vi "SP_Breakdown Summery DayWisewise.vi"() -> ()   [LabVIEW 2017]
uses:
  <vilib>/Math Plots/3D Math Plots/3D Pie/3D Pie XCtrl/3D Pie.xctl
  <vilib>/addons/database/Connection.llb/DB Tools Open Connec (Path).vi
  <vilib>/Math Plots/3D Math Plots/3D Pie/3D Pie Datatype/Public/Plot Helper (Vector).vi
  <vilib>/addons/database/NI_Database_API.lvlib
  <vilib>/Math Plots/3D Math Plots/3D Pie/3D Pie Datatype/3D Pie Datatype.lvclass
panel:
  out "error out 2":errorcluster
  out "Boolean":bool
  in  "Cancel Button - Archive":bool
  in  "Get Rport 2":bool
  in  "Download 2":bool
  in  "error in":errorcluster
  in  "To":timestamp format="%<%Y-%m-%d>T"
  in  "From":timestamp format="%<%Y-%m-%d>T"
  out "error out":errorcluster
  out "O/P 4":string[](array[string])
  out "month":string
  out "Count":string[](array[string])
  out "Station ID":string[](array[string])
  out "Count out":string[](array[string])
  out "Elements Found out":string[](array[string])
  in  "stop":bool
  in  "Select Station":string(combo)
  in  "Shift":string(combo)
  out "T":string
  out "SS":string
  out "Q":string
  out "Maint":string
  out "Mat":string
  out "S":string
  in  "Select Year":string(combo)
  in  "Select Month":string(combo)
  in  "Tab Control":T1(tab)
  out "Table Control":string[][](table)
  out "heading 6":string="Total"
  out "heading 5":string="Production"
  out "heading 4":string="Qaulity"
  out "heading 3":string="Maintenance"
  out "heading2":string="Logistics"
  out "heading 1":string="Gap Leader"
  out "Count":refnum<class "3D Plot Datatype.lvclass">[](xcontrol)
  out "Duration":refnum<class "3D Plot Datatype.lvclass">[](xcontrol)
  # "Breakdown Summary Report (Day Wise)"
  # "S"
  # "M"
  # "TT"
  # "M"
  # "Q"
  # "SS"
  # "Designed And Developed By - Infinity Automation Systems Pvt. Ltd."
  # "Material"
  # "Date"
  # "Maintenance"
  # "Quality"
  # "Startup/Setup"
  # "Total"
  # "Safety"
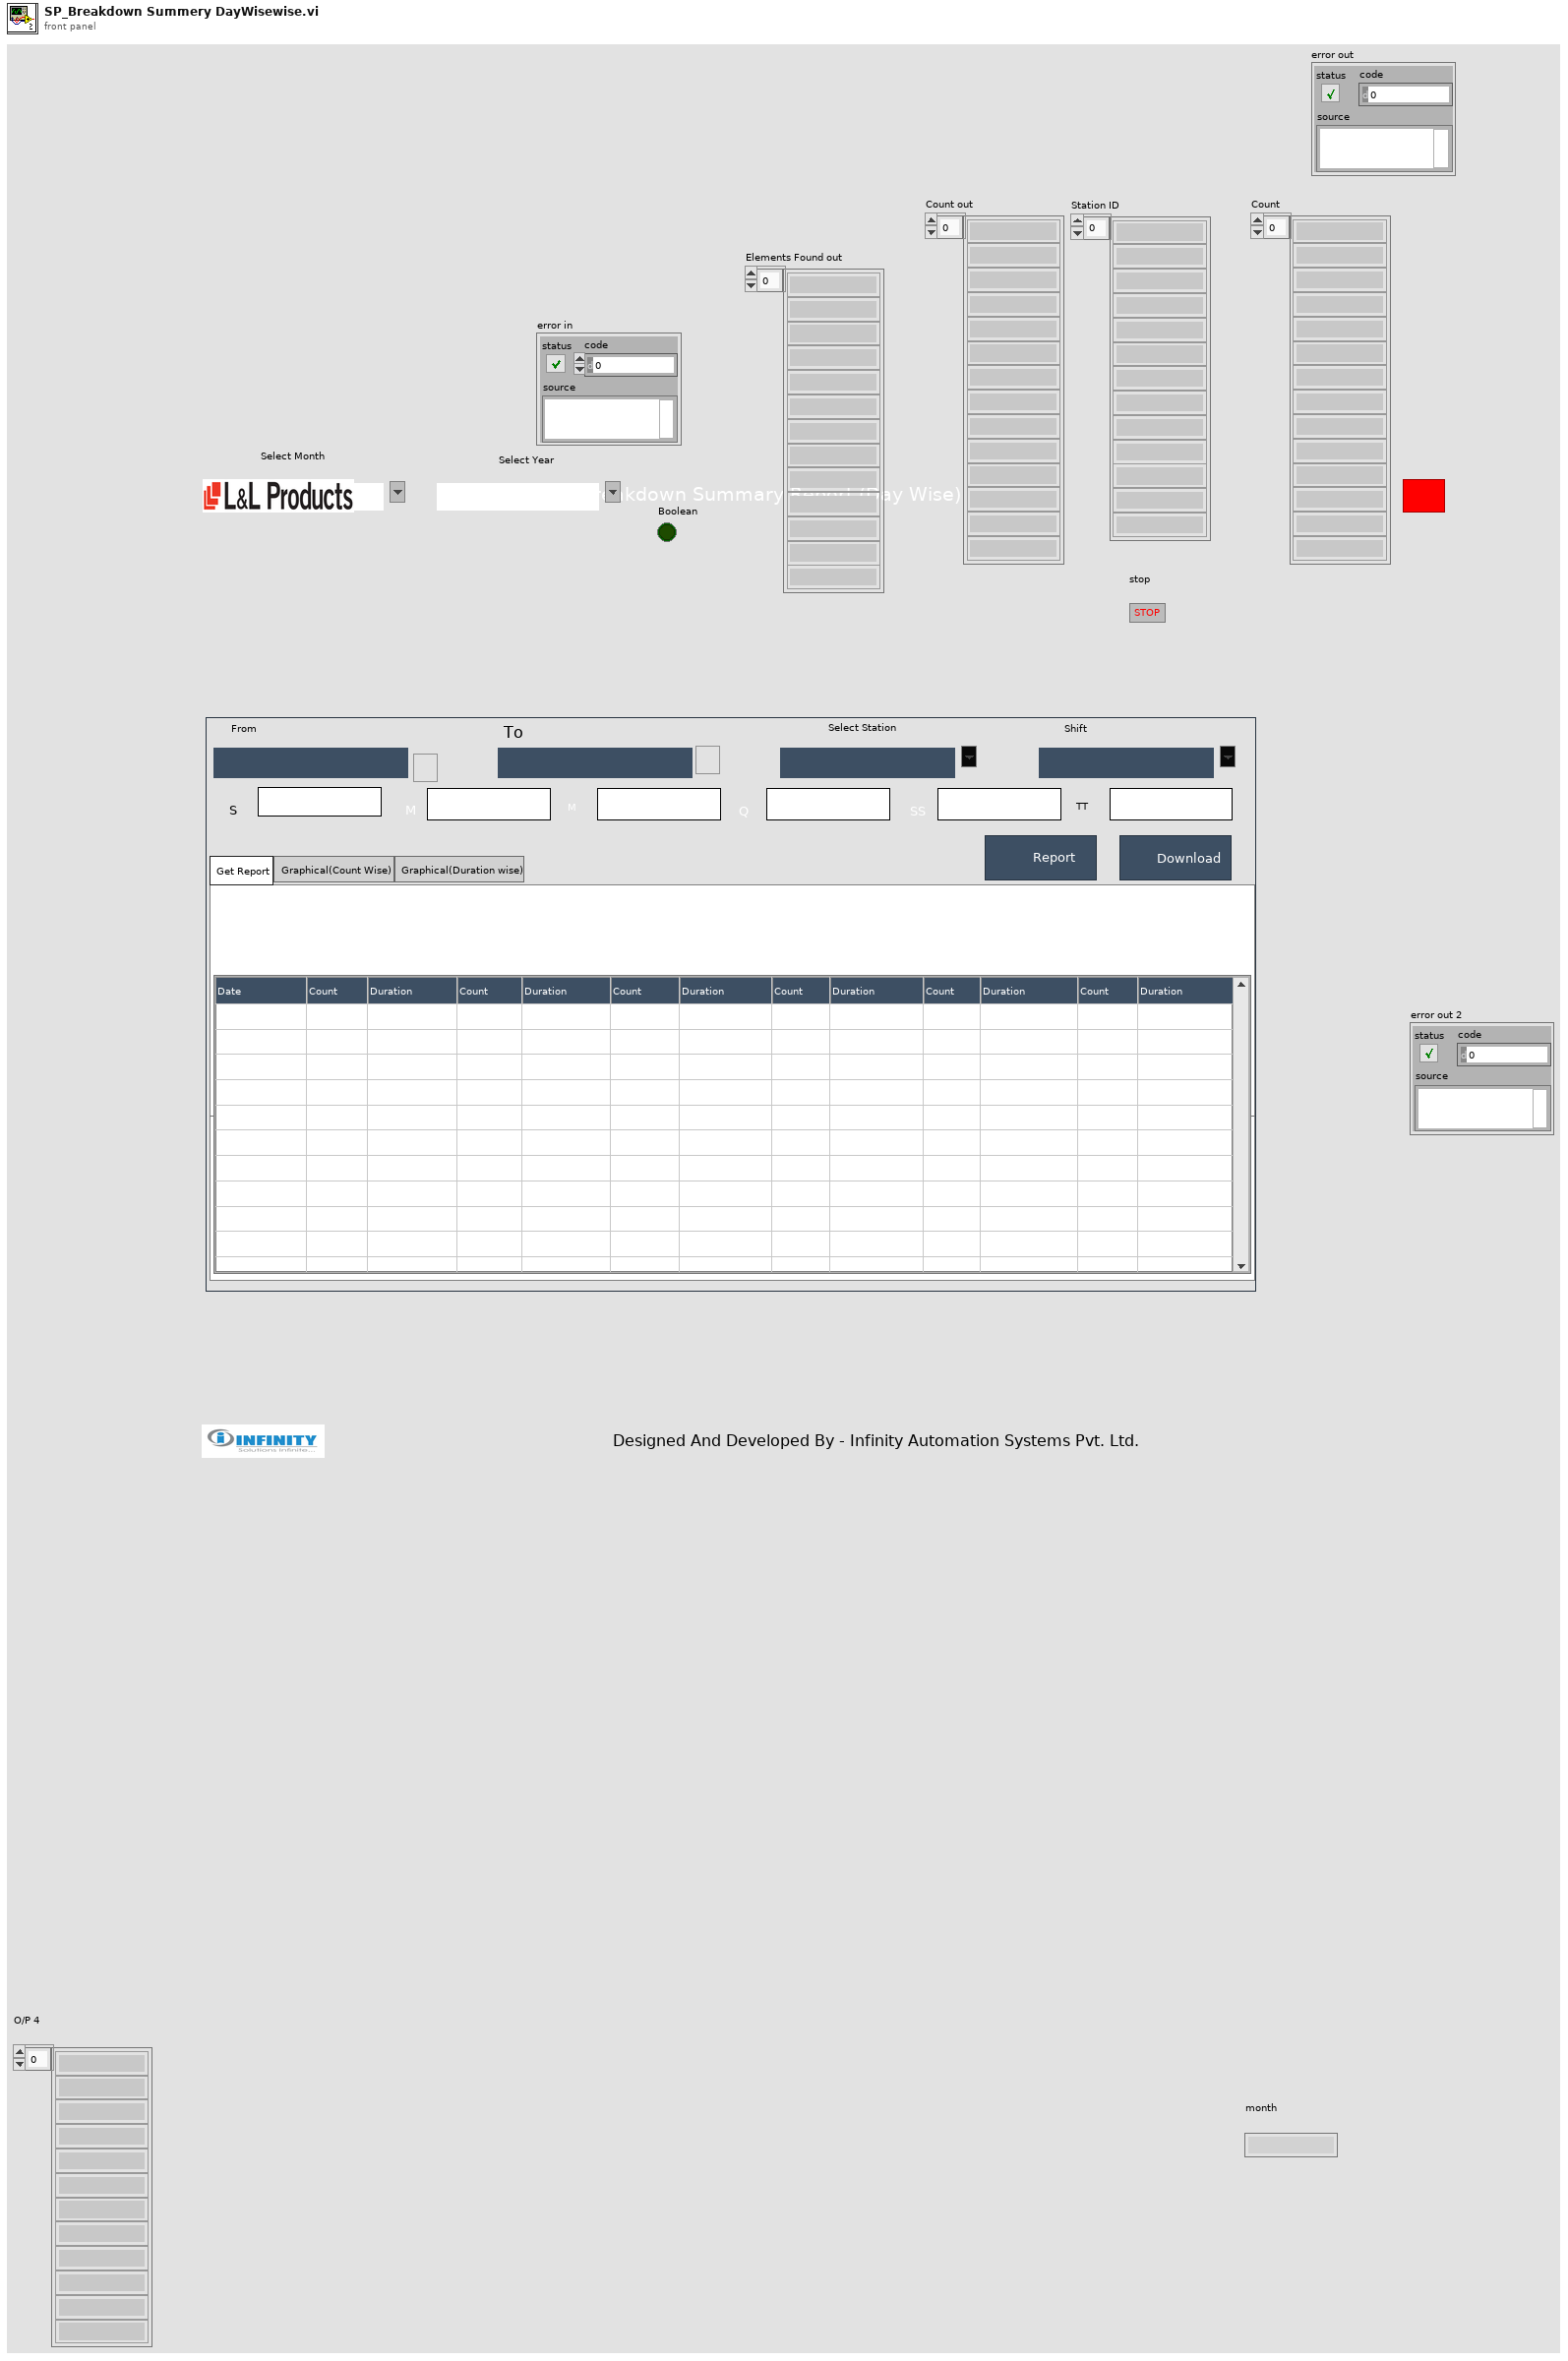
[diagram p1: front panel]
types:
  T1 = enum32{"Get Report", "Graphical(Count Wise) ", "Graphical(Duration wise)"}
  T2 = typedef "NI_Database_API.lvlib/Conn ObjectReference.ctl" = refnum<k1>
  T3 = enum32{"invalid app kind", "Development System", "Run Time System", "Student Edition", "Embedded LabVIEW", "Evaluation", "Custom"}
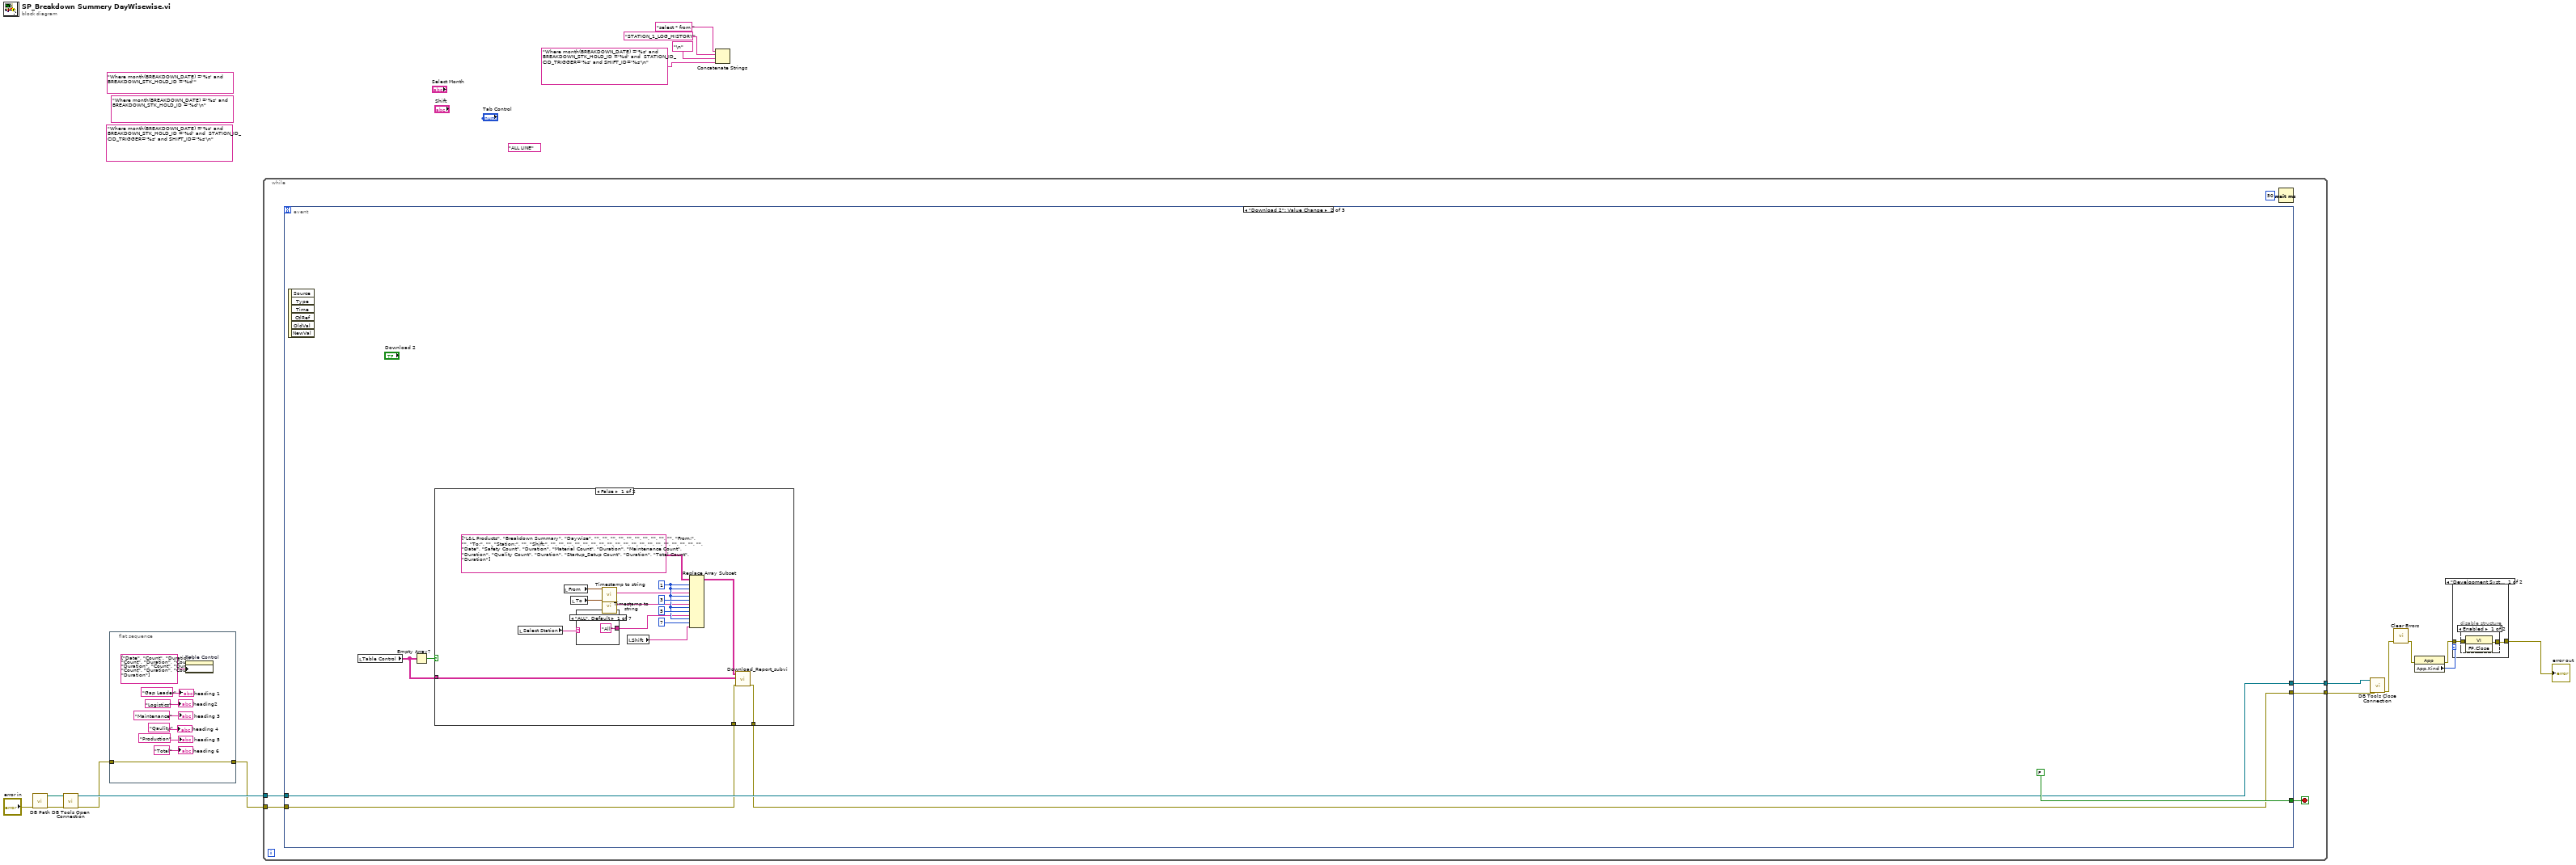
[diagram p0: block diagram]
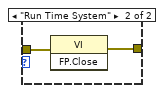
[diagram p3: hidden frame]
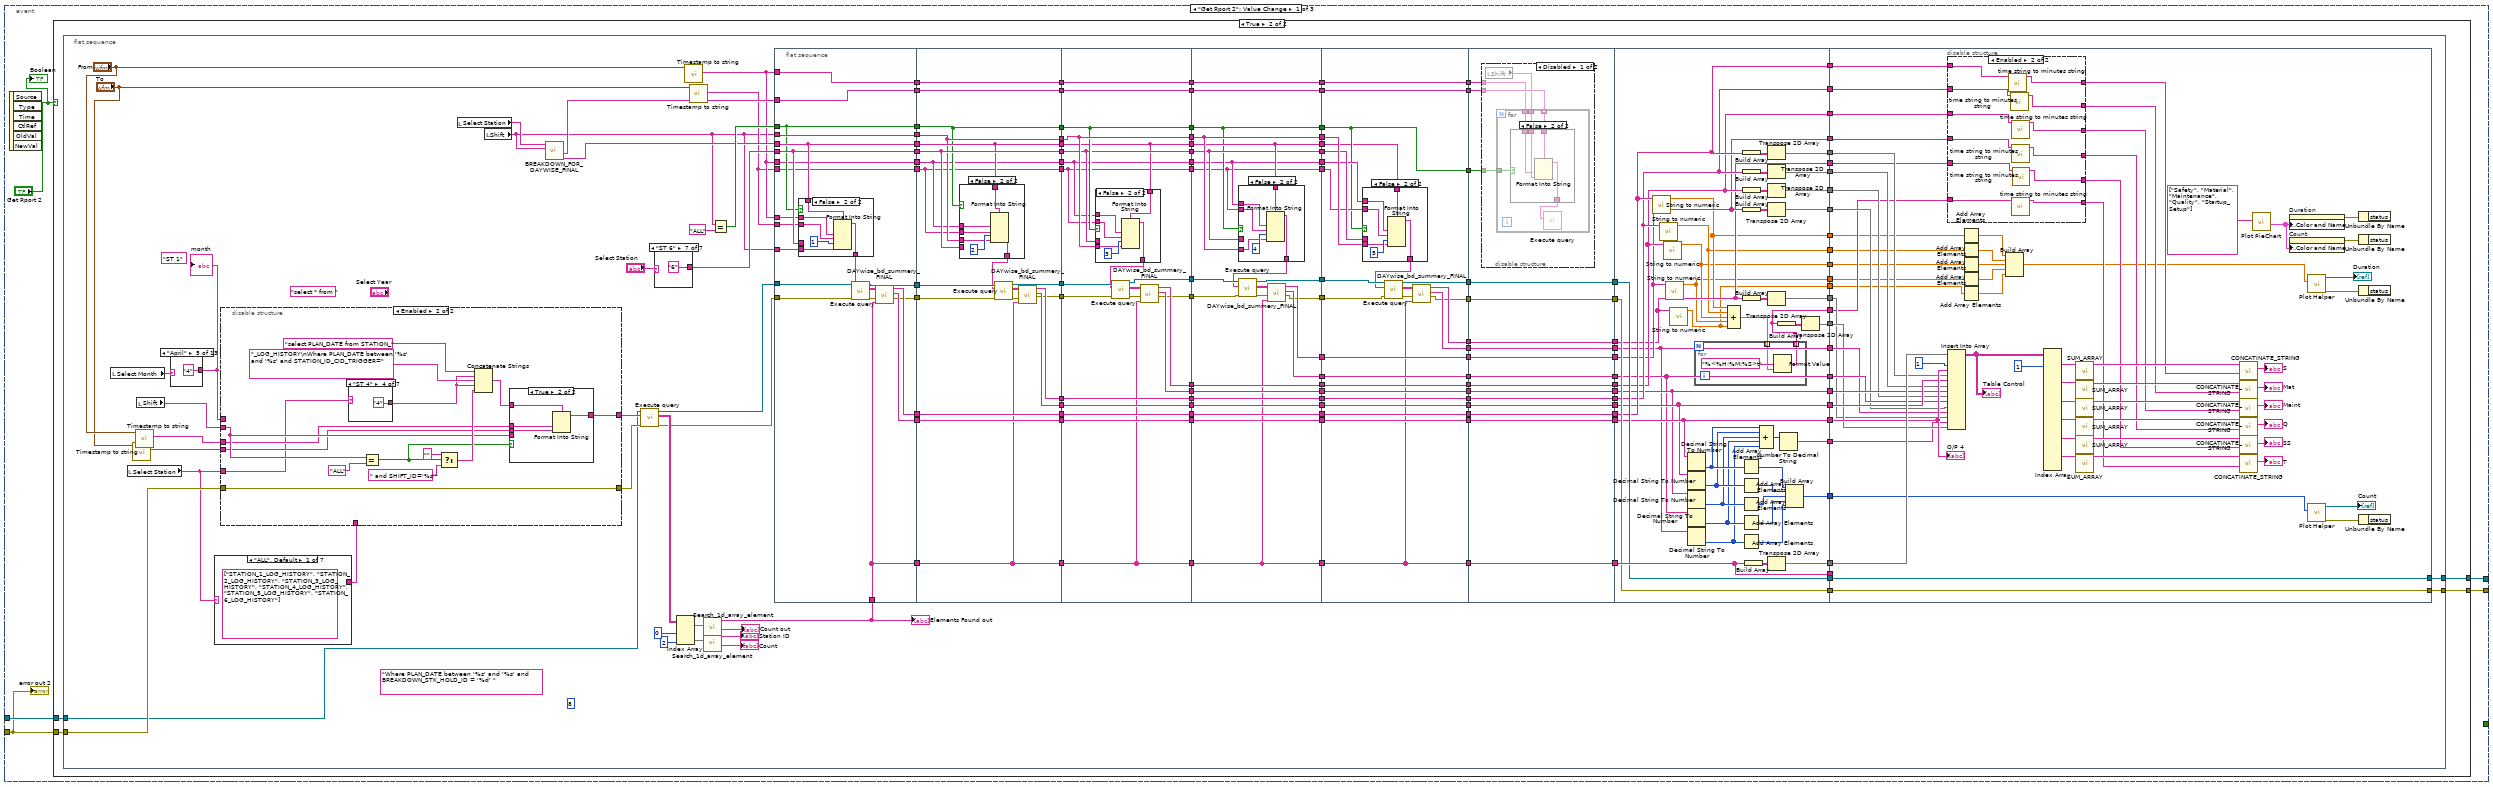
[diagram p4: hidden frame]
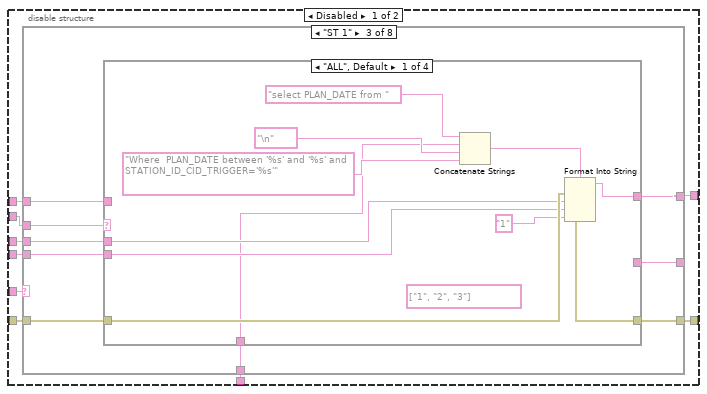
[diagram p6: hidden frame]
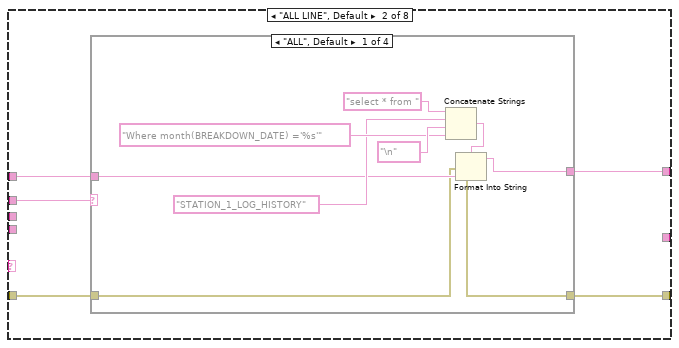
[diagram p8: hidden frame]
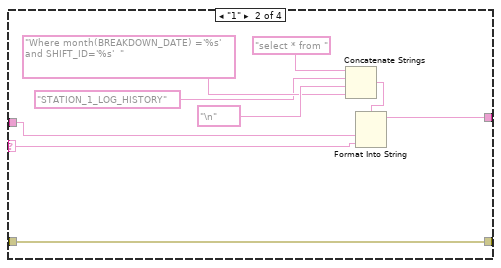
[diagram p9: hidden frame]
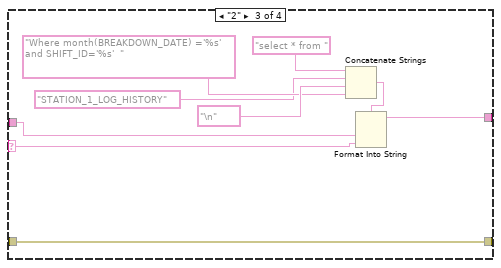
[diagram p10: hidden frame]
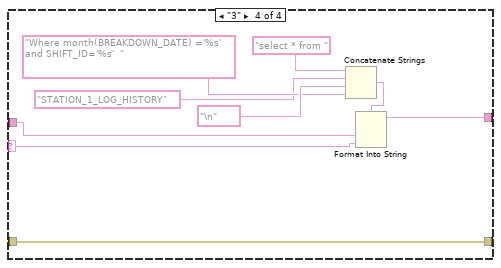
[diagram p11: hidden frame]
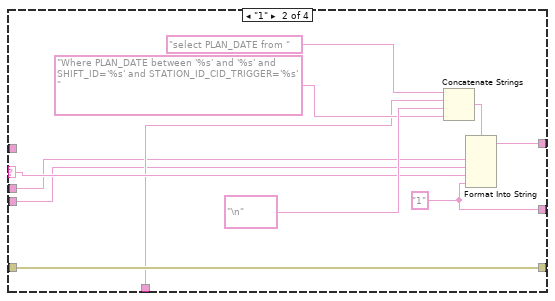
[diagram p12: hidden frame]
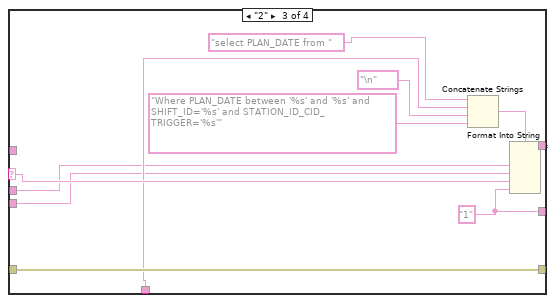
[diagram p13: hidden frame]
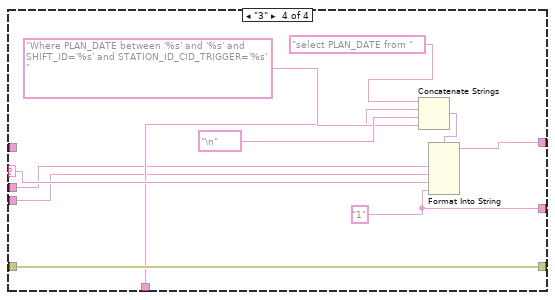
[diagram p14: hidden frame]
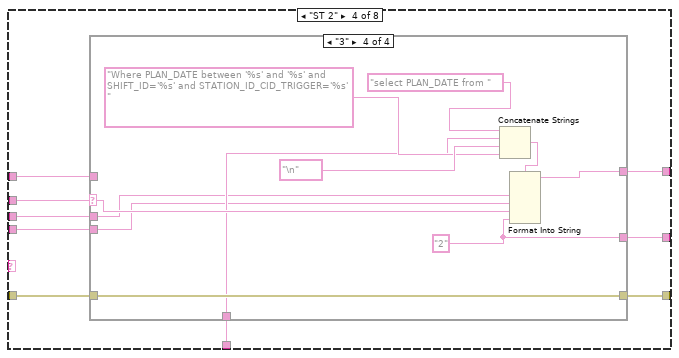
[diagram p15: hidden frame]
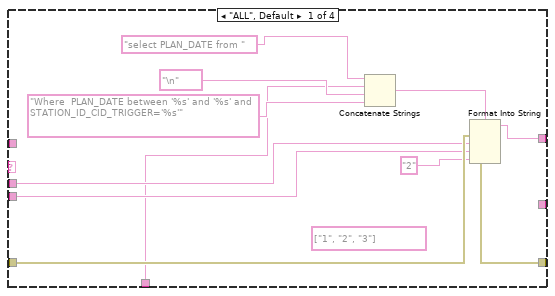
[diagram p16: hidden frame]
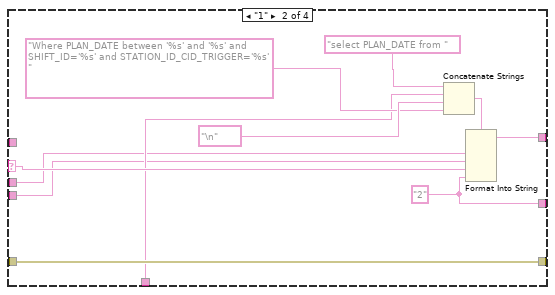
[diagram p17: hidden frame]
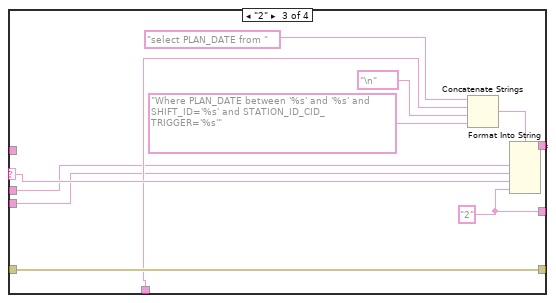
[diagram p18: hidden frame]
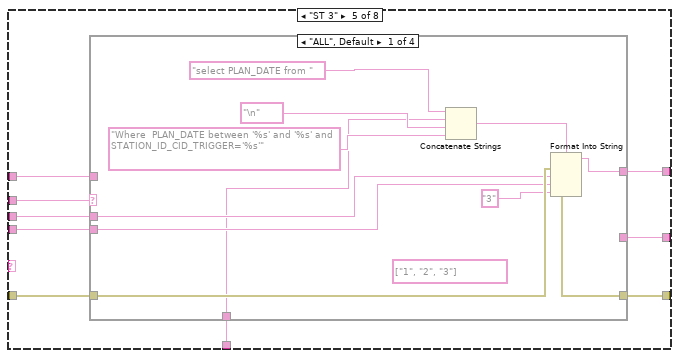
[diagram p19: hidden frame]
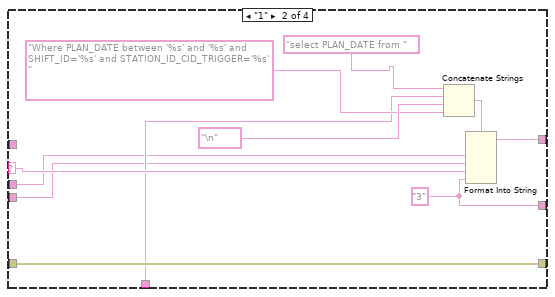
[diagram p20: hidden frame]
diagram:
  (unwired) "Where month(BREAKDOWN_DATE) ='%s' and  BREAKDOWN_STK_HOLD_ID ='%d' and  STATION_ID_CID_TRIGGER='%s' and SHIFT_ID='%s'\n" ("condition")
  (unwired) "Where month(BREAKDOWN_DATE) ='%s' and  BREAKDOWN_STK_HOLD_ID ='%d'" ("condition")
  (unwired) "Where month(BREAKDOWN_DATE) ='%s' and  BREAKDOWN_STK_HOLD_ID ='%d'\n" ("condition")
  (unwired) "ALL LINE" ("Select Line 2")
  n1 = call "DB Path.vi"("error in"="error in") -> ("error out"=w17:errorcluster, "DB Path"=w16:path)  [unwired: 9 in]
  n2 = call-poly <vilib>:"DB Tools Open Connection.vi"("error in (no error)"=w17, "connection information"=w16) -> ("error out"=w2:errorcluster, "connection reference"=w15:T2)  [unwired: 6 in]
  n3 = flat-sequence {
    tunnel: [w18] -> w1
    tunnel: w2 -> [w18]
    frame #0 {
      n4 = property on="Table Control" class="Tbl (strict)"("Column Headers[]"=string[] ["Date", "Count", "Duration", "Count", "Duration", "Count", "Duration", "Count", "Duration", "Count", "Duration", "Count", "Duration"] ("Column Header Strings[]")) -> ()  [unwired: 2 in, 2 out]
      "heading 1" <- "Gap Leader" ("heading 1")
      "heading2" <- "Logistics" ("heading2")
      "heading 3" <- "Maintenance" ("heading 3")
      "heading 4" <- "Qaulity" ("heading 4")
      "heading 5" <- "Production" ("heading 5")
      "heading 6" <- "Total" ("heading 6")
    }
  }
  n5 = while {
    tunnel: w1 -> [w31]
    tunnel: w15 -> [w30]
    tunnel: [w28] -> w5
    tunnel: [w27] -> w6
    stop <- w29 stop-if-true
    n6 = event shown="[1] \"Download 2\": Value Change" {
      selector: _ -> [_ _ _]
      dyn-events: _ -> [_ _ _]
      timeout: _ -> [_ _ _]
      tunnel: w31 -> [w33 w985 w1014]
      tunnel: w30 -> [w36 w986 w1013]
      tunnel: [_ FALSE ("Cancel Button - Archive") "Cancel Button - Archive"] -> w29
      tunnel: [w35 w984 w1014] -> w28
      tunnel: [w34 w986 w1013] -> w27
      event "Get Rport 2": Value Change {
        n7 = event-data() -> ()  [unwired: 1 in, 6 out]
        n8 = case shown="True" "Get Rport 2" {
          tunnel: w33 -> [_ w40]
          tunnel: w36 -> [_ w39]
          tunnel: [_ w38] -> w35
          tunnel: [_ w37] -> w34
          frame False {
          }
          frame True {
            n9 = flat-sequence {
              tunnel: w40 -> [w193]
              tunnel: w39 -> [w120]
              tunnel: [w118] -> w38
              tunnel: [w116] -> w37
              frame #0 {
                (unwired) "select * from " ("string")
                (unwired) 8 ("disabled index (col)")
                (unwired) "Where PLAN_DATE between '%s' and '%s' and BREAKDOWN_STK_HOLD_ID = '%d' "
                (unwired) "ST 1" ("Select Station")
                n10 = local read "Select Month"() -> (w190:string)
                n11 = local read "Select Station"() -> (w112:string)
                n12 = call "Timestamp to string.vi"("time stamp"="To") -> ("Date"=w52:string)  [unwired: 8 in, 2 out]
                n13 = call "Timestamp to string.vi"("time stamp"="From") -> ("Date"=w53:string)  [unwired: 8 in, 2 out]
                n14 = local read "Shift"() -> (w100:string)
                n15 = case shown="\"April\"" w190 {
                  tunnel: ["1" "1" "2" "3" "4" "5" "6" "7" "8" "9" "10" "11" "12"] -> w119
                  frame "False", Default {
                  }
                  frame "January" {
                  }
                  frame "February" {
                  }
                  frame "March" {
                  }
                  frame "April" {
                  }
                  frame "May" {
                  }
                  frame "June" {
                  }
                  frame "July" {
                  }
                  frame "August" {
                  }
                  frame "September" {
                  }
                  frame "October" {
                  }
                  frame "November" {
                  }
                  frame "December" {
                  }
                }
                "month" <- w119
                n16 = case shown="\"ALL\", Default" w112 {
                  tunnel: [_ "STATION_1_LOG_HISTORY" "STATION_2_LOG_HISTORY" ("table") "STATION_3_LOG_HISTORY" ("table") "STATION_4_LOG_HISTORY" ("table") "STATION_5_LOG_HISTORY" ("table") "STATION_6_LOG_HISTORY" ("table")] -> w99
                  frame "ALL", Default {
                    (unwired) string[] ["STATION_1_LOG_HISTORY", "STATION_2_LOG_HISTORY", "STATION_3_LOG_HISTORY", "STATION_4_LOG_HISTORY", "STATION_5_LOG_HISTORY", "STATION_6_LOG_HISTORY"]
                  }
                  frame "ST 1" {
                  }
                  frame "ST 2" {
                  }
                  frame "ST 3" {
                  }
                  frame "ST 4" {
                  }
                  frame "ST 5" {
                  }
                  frame "ST 6" {
                  }
                }
                n17 = disable-structure shown="Enabled" {
                  disable-tunnel: [w206 w571] -> w197
                  disable-tunnel: w193 -> [w205 w567]
                  disable-tunnel: [w204 w567] -> w192
                  disable-tunnel: w119 -> [w203 _]
                  disable-tunnel: w112 -> [w202 w566]
                  disable-tunnel: w100 -> [w201 w570]
                  disable-tunnel: w99 -> [w200 _]
                  disable-tunnel: w53 -> [w199 w569]
                  disable-tunnel: w52 -> [w198 w568]
                  frame Disabled {
                    n18 = case shown="\"ST 1\"" w202 {
                      tunnel: w203 -> [_ w211 w256 w309 w362 w415 w468 w521]
                      tunnel: [_ w210 w255 w308 w361 w414 w467 w520] -> w206
                      tunnel: w205 -> [_ w209 w254 w307 w360 w413 w466 w519]
                      tunnel: [_ w208 w253 w306 w359 w412 w465 w518] -> w204
                      tunnel: [_ _ w252 w305 w358 w411 w464 w517] -> _
                      tunnel: w199 -> [_ _ w251 w304 w357 w410 w463 w516]
                      tunnel: w198 -> [_ _ w250 w303 w356 w409 w462 w515]
                      tunnel: w201 -> [_ w207 w248 w301 w354 w407 w460 w513]
                      tunnel: w200 -> [_ _ w249 w302 w355 w408 w461 w514]
                      frame "False" {
                      }
                      frame "ALL LINE", Default {
                        n19 = case shown="\"ALL\", Default" w207 {
                          selector: w207 -> [_ w222 w231 w240]
                          tunnel: [w216 w225 w234 w243] -> w210
                          tunnel: [w215 w221 w230 w239] -> w208
                          tunnel: w211 -> [w213 w223 w232 w241]
                          tunnel: w209 -> [w212 w221 w230 w239]
                          frame "ALL", Default {
                            n20 = Concatenate Strings("select * from " ("string"), "STATION_1_LOG_HISTORY" ("table"), "\n" ("string"), "Where month(BREAKDOWN_DATE) ='%s'" ("condition")) -> (w217:string)
                            n21 = Format Into String(format string=w217, error in=w212, w213) -> (resulting string=w216:string, error out=w215:errorcluster)  [unwired: 1 in]
                          }
                          frame "1" {
                            n22 = Concatenate Strings("select * from " ("string"), "STATION_1_LOG_HISTORY" ("table"), "\n" ("string"), "Where month(BREAKDOWN_DATE) ='%s' and SHIFT_ID='%s'  " ("condition")) -> (w227:string)
                            n23 = Format Into String(format string=w227, w223, w222) -> (resulting string=w225:string)  [unwired: 2 in, 1 out]
                          }
                          frame "2" {
                            n24 = Concatenate Strings("select * from " ("string"), "STATION_1_LOG_HISTORY" ("table"), "\n" ("string"), "Where month(BREAKDOWN_DATE) ='%s' and SHIFT_ID='%s'  " ("condition")) -> (w236:string)
                            n25 = Format Into String(format string=w236, w232, w231) -> (resulting string=w234:string)  [unwired: 2 in, 1 out]
                          }
                          frame "3" {
                            n26 = Concatenate Strings("select * from " ("string"), "STATION_1_LOG_HISTORY" ("table"), "\n" ("string"), "Where month(BREAKDOWN_DATE) ='%s' and SHIFT_ID='%s'  " ("condition")) -> (w245:string)
                            n27 = Format Into String(format string=w245, w241, w240) -> (resulting string=w243:string)  [unwired: 2 in, 1 out]
                          }
                        }
                      }
                      frame "ST 1" {
                        n28 = case shown="\"ALL\", Default" w248 {
                          selector: w248 -> [_ w275 w286 w297]
                          tunnel: [w263 w276 w287 w298] -> w255
                          tunnel: [w262 w274 w285 w296] -> w253
                          tunnel: w256 -> [_ _ _ _]
                          tunnel: w254 -> [w261 w274 w285 w296]
                          tunnel: [_ w272 w283 w294] -> w252
                          tunnel: w251 -> [w259 w270 w281 w292]
                          tunnel: w250 -> [w258 w269 w280 w291]
                          tunnel: w249 -> [w257 w271 w282 w293]
                          frame "ALL", Default {
                            (unwired) string[] ["1", "2", "3"]
                            n29 = Concatenate Strings("select PLAN_DATE from " ("string"), w257, "\n" ("string"), "Where  PLAN_DATE between '%s' and '%s' and  STATION_ID_CID_TRIGGER='%s'" ("condition")) -> (w264:string)
                            n30 = Format Into String(format string=w264, error in=w261, w259, w258, "1") -> (resulting string=w263:string, error out=w262:errorcluster)  [unwired: 1 in]
                          }
                          frame "1" {
                            w272 = "1"
                            n31 = Concatenate Strings("select PLAN_DATE from " ("string"), w271, "\n" ("string"), "Where PLAN_DATE between '%s' and '%s' and SHIFT_ID='%s' and STATION_ID_CID_TRIGGER='%s'   " ("condition")) -> (w273:string)
                            n32 = Format Into String(format string=w273, w270, w269, w275, w272) -> (resulting string=w276:string)  [unwired: 2 in, 1 out]
                          }
                          frame "2" {
                            w283 = "1" ("input 3")
                            n33 = Concatenate Strings("select PLAN_DATE from " ("string"), w282, "\n" ("string"), "Where PLAN_DATE between '%s' and '%s' and SHIFT_ID='%s' and STATION_ID_CID_TRIGGER='%s'" ("condition")) -> (w288:string)
                            n34 = Format Into String(format string=w288, w281, w280, w286, w283) -> (resulting string=w287:string)  [unwired: 2 in, 1 out]
                          }
                          frame "3" {
                            w294 = "1" ("input 3")
                            n35 = Concatenate Strings("select PLAN_DATE from " ("string"), w293, "\n" ("string"), "Where PLAN_DATE between '%s' and '%s' and SHIFT_ID='%s' and STATION_ID_CID_TRIGGER='%s'   " ("condition")) -> (w299:string)
                            n36 = Format Into String(format string=w299, w292, w291, w297, w294) -> (resulting string=w298:string)  [unwired: 2 in, 1 out]
                          }
                        }
                      }
                      frame "ST 2" {
                        n37 = case shown="\"3\"" w301 {
                          selector: w301 -> [_ w328 w339 w350]
                          tunnel: [w317 w329 w340 w351] -> w308
                          tunnel: [w316 w327 w338 w349] -> w306
                          tunnel: w309 -> [_ _ _ _]
                          tunnel: w307 -> [w315 w327 w338 w349]
                          tunnel: [_ w325 w336 w347] -> w305
                          tunnel: w304 -> [w313 w323 w334 w345]
                          tunnel: w303 -> [w312 w322 w333 w344]
                          tunnel: w302 -> [w311 w324 w335 w346]
                          frame "ALL", Default {
                            (unwired) string[] ["1", "2", "3"]
                            n38 = Concatenate Strings("select PLAN_DATE from " ("string"), w311, "\n" ("string"), "Where  PLAN_DATE between '%s' and '%s' and  STATION_ID_CID_TRIGGER='%s'" ("condition")) -> (w318:string)
                            n39 = Format Into String(format string=w318, error in=w315, w313, w312, "2") -> (resulting string=w317:string, error out=w316:errorcluster)  [unwired: 1 in]
                          }
                          frame "1" {
                            w325 = "2"
                            n40 = Concatenate Strings("select PLAN_DATE from " ("string"), w324, "\n" ("string"), "Where PLAN_DATE between '%s' and '%s' and SHIFT_ID='%s' and STATION_ID_CID_TRIGGER='%s'   " ("condition")) -> (w326:string)
                            n41 = Format Into String(format string=w326, w323, w322, w328, w325) -> (resulting string=w329:string)  [unwired: 2 in, 1 out]
                          }
                          frame "2" {
                            w336 = "2" ("input 3")
                            n42 = Concatenate Strings("select PLAN_DATE from " ("string"), w335, "\n" ("string"), "Where PLAN_DATE between '%s' and '%s' and SHIFT_ID='%s' and STATION_ID_CID_TRIGGER='%s'" ("condition")) -> (w341:string)
                            n43 = Format Into String(format string=w341, w334, w333, w339, w336) -> (resulting string=w340:string)  [unwired: 2 in, 1 out]
                          }
                          frame "3" {
                            w347 = "2" ("input 3")
                            n44 = Concatenate Strings("select PLAN_DATE from " ("string"), w346, "\n" ("string"), "Where PLAN_DATE between '%s' and '%s' and SHIFT_ID='%s' and STATION_ID_CID_TRIGGER='%s'   " ("condition")) -> (w352:string)
                            n45 = Format Into String(format string=w352, w345, w344, w350, w347) -> (resulting string=w351:string)  [unwired: 2 in, 1 out]
                          }
                        }
                      }
                      frame "ST 3" {
                        n46 = case shown="\"ALL\", Default" w354 {
                          selector: w354 -> [_ w381 w392 w403]
                          tunnel: [w370 w382 w393 w404] -> w361
                          tunnel: [w369 w380 w391 w402] -> w359
                          tunnel: w362 -> [_ _ _ _]
                          tunnel: w360 -> [w368 w380 w391 w402]
                          tunnel: [_ w378 w389 w400] -> w358
                          tunnel: w357 -> [w366 w376 w387 w398]
                          tunnel: w356 -> [w365 w375 w386 w397]
                          tunnel: w355 -> [w364 w377 w388 w399]
                          frame "ALL", Default {
                            (unwired) string[] ["1", "2", "3"]
                            n47 = Concatenate Strings("select PLAN_DATE from " ("string"), w364, "\n" ("string"), "Where  PLAN_DATE between '%s' and '%s' and  STATION_ID_CID_TRIGGER='%s'" ("condition")) -> (w371:string)
                            n48 = Format Into String(format string=w371, error in=w368, w366, w365, "3") -> (resulting string=w370:string, error out=w369:errorcluster)  [unwired: 1 in]
                          }
                          frame "1" {
                            w378 = "3"
                            n49 = Concatenate Strings("select PLAN_DATE from " ("string"), w377, "\n" ("string"), "Where PLAN_DATE between '%s' and '%s' and SHIFT_ID='%s' and STATION_ID_CID_TRIGGER='%s'   " ("condition")) -> (w379:string)
                            n50 = Format Into String(format string=w379, w376, w375, w381, w378) -> (resulting string=w382:string)  [unwired: 2 in, 1 out]
                          }
                          frame "2" {
                            w389 = "3" ("input 3")
                            n51 = Concatenate Strings("select PLAN_DATE from " ("string"), w388, "\n" ("string"), "Where PLAN_DATE between '%s' and '%s' and SHIFT_ID='%s' and STATION_ID_CID_TRIGGER='%s'" ("condition")) -> (w394:string)
                            n52 = Format Into String(format string=w394, w387, w386, w392, w389) -> (resulting string=w393:string)  [unwired: 2 in, 1 out]
                          }
                          frame "3" {
                            w400 = "3" ("input 3")
                            n53 = Concatenate Strings("select PLAN_DATE from " ("string"), w399, "\n" ("string"), "Where PLAN_DATE between '%s' and '%s' and SHIFT_ID='%s' and STATION_ID_CID_TRIGGER='%s'   " ("condition")) -> (w405:string)
                            n54 = Format Into String(format string=w405, w398, w397, w403, w400) -> (resulting string=w404:string)  [unwired: 2 in, 1 out]
                          }
                        }
                      }
                      frame "ST 4" {
                        n55 = case shown="\"3\"" w407 {
                          selector: w407 -> [_ w434 w445 w456]
                          tunnel: [w423 w435 w446 w457] -> w414
                          tunnel: [w422 w433 w444 w455] -> w412
                          tunnel: w415 -> [_ _ _ _]
                          tunnel: w413 -> [w421 w433 w444 w455]
                          tunnel: [_ w431 w442 w453] -> w411
                          tunnel: w410 -> [w419 w429 w440 w451]
                          tunnel: w409 -> [w418 w428 w439 w450]
                          tunnel: w408 -> [w417 w430 w441 w452]
                          frame "ALL", Default {
                            (unwired) string[] ["1", "2", "3"]
                            n56 = Concatenate Strings("select PLAN_DATE from " ("string"), w417, "\n" ("string"), "Where  PLAN_DATE between '%s' and '%s' and  STATION_ID_CID_TRIGGER='%s'" ("condition")) -> (w424:string)
                            n57 = Format Into String(format string=w424, error in=w421, w419, w418, "4") -> (resulting string=w423:string, error out=w422:errorcluster)  [unwired: 1 in]
                          }
                          frame "1" {
                            w431 = "4"
                            n58 = Concatenate Strings("select PLAN_DATE from " ("string"), w430, "\n" ("string"), "Where PLAN_DATE between '%s' and '%s' and SHIFT_ID='%s' and STATION_ID_CID_TRIGGER='%s'   " ("condition")) -> (w432:string)
                            n59 = Format Into String(format string=w432, w429, w428, w434, w431) -> (resulting string=w435:string)  [unwired: 2 in, 1 out]
                          }
                          frame "2" {
                            w442 = "4" ("input 3")
                            n60 = Concatenate Strings("select PLAN_DATE from " ("string"), w441, "\n" ("string"), "Where PLAN_DATE between '%s' and '%s' and SHIFT_ID='%s' and STATION_ID_CID_TRIGGER='%s'" ("condition")) -> (w447:string)
                            n61 = Format Into String(format string=w447, w440, w439, w445, w442) -> (resulting string=w446:string)  [unwired: 2 in, 1 out]
                          }
                          frame "3" {
                            w453 = "4" ("input 3")
                            n62 = Concatenate Strings("select PLAN_DATE from " ("string"), w452, "\n" ("string"), "Where PLAN_DATE between '%s' and '%s' and SHIFT_ID='%s' and STATION_ID_CID_TRIGGER='%s'   " ("condition")) -> (w458:string)
                            n63 = Format Into String(format string=w458, w451, w450, w456, w453) -> (resulting string=w457:string)  [unwired: 2 in, 1 out]
                          }
                        }
                      }
                      frame "ST 5" {
                        n64 = case shown="\"1\"" w460 {
                          selector: w460 -> [_ w487 w498 w509]
                          tunnel: [w476 w488 w499 w510] -> w467
                          tunnel: [w475 w486 w497 w508] -> w465
                          tunnel: w468 -> [_ _ _ _]
                          tunnel: w466 -> [w474 w486 w497 w508]
                          tunnel: [_ w484 w495 w506] -> w464
                          tunnel: w463 -> [w472 w482 w493 w504]
                          tunnel: w462 -> [w471 w481 w492 w503]
                          tunnel: w461 -> [w470 w483 w494 w505]
                          frame "ALL", Default {
                            (unwired) string[] ["1", "2", "3"]
                            n65 = Concatenate Strings("select PLAN_DATE from " ("string"), w470, "\n" ("string"), "Where  PLAN_DATE between '%s' and '%s' and  STATION_ID_CID_TRIGGER='%s'" ("condition")) -> (w477:string)
                            n66 = Format Into String(format string=w477, error in=w474, w472, w471, "5") -> (resulting string=w476:string, error out=w475:errorcluster)  [unwired: 1 in]
                          }
                          frame "1" {
                            w484 = "5"
                            n67 = Concatenate Strings("select PLAN_DATE from " ("string"), w483, "\n" ("string"), "Where PLAN_DATE between '%s' and '%s' and SHIFT_ID='%s' and STATION_ID_CID_TRIGGER='%s'   " ("condition")) -> (w485:string)
                            n68 = Format Into String(format string=w485, w482, w481, w487, w484) -> (resulting string=w488:string)  [unwired: 2 in, 1 out]
                          }
                          frame "2" {
                            w495 = "5" ("input 3")
                            n69 = Concatenate Strings("select PLAN_DATE from " ("string"), w494, "\n" ("string"), "Where PLAN_DATE between '%s' and '%s' and SHIFT_ID='%s' and STATION_ID_CID_TRIGGER='%s'" ("condition")) -> (w500:string)
                            n70 = Format Into String(format string=w500, w493, w492, w498, w495) -> (resulting string=w499:string)  [unwired: 2 in, 1 out]
                          }
                          frame "3" {
                            w506 = "5" ("input 3")
                            n71 = Concatenate Strings("select PLAN_DATE from " ("string"), w505, "\n" ("string"), "Where PLAN_DATE between '%s' and '%s' and SHIFT_ID='%s' and STATION_ID_CID_TRIGGER='%s'   " ("condition")) -> (w511:string)
                            n72 = Format Into String(format string=w511, w504, w503, w509, w506) -> (resulting string=w510:string)  [unwired: 2 in, 1 out]
                          }
                        }
                      }
                      frame "ST 6" {
                        n73 = case shown="\"1\"" w513 {
                          selector: w513 -> [_ w540 w551 w562]
                          tunnel: [w529 w541 w552 w563] -> w520
                          tunnel: [w528 w539 w550 w561] -> w518
                          tunnel: w521 -> [_ _ _ _]
                          tunnel: w519 -> [w527 w539 w550 w561]
                          tunnel: [_ w537 w548 w559] -> w517
                          tunnel: w516 -> [w525 w535 w546 w557]
                          tunnel: w515 -> [w524 w534 w545 w556]
                          tunnel: w514 -> [w523 w536 w547 w558]
                          frame "ALL", Default {
                            (unwired) string[] ["1", "2", "3"]
                            n74 = Concatenate Strings("select PLAN_DATE from " ("string"), w523, "\n" ("string"), "Where  PLAN_DATE between '%s' and '%s' and  STATION_ID_CID_TRIGGER='%s'" ("condition")) -> (w530:string)
                            n75 = Format Into String(format string=w530, error in=w527, w525, w524, "6") -> (resulting string=w529:string, error out=w528:errorcluster)  [unwired: 1 in]
                          }
                          frame "1" {
                            w537 = "6"
                            n76 = Concatenate Strings("select PLAN_DATE from " ("string"), w536, "\n" ("string"), "Where PLAN_DATE between '%s' and '%s' and SHIFT_ID='%s' and STATION_ID_CID_TRIGGER='%s'   " ("condition")) -> (w538:string)
                            n77 = Format Into String(format string=w538, w535, w534, w540, w537) -> (resulting string=w541:string)  [unwired: 2 in, 1 out]
                          }
                          frame "2" {
                            w548 = "6" ("input 3")
                            n78 = Concatenate Strings("select PLAN_DATE from " ("string"), w547, "\n" ("string"), "Where PLAN_DATE between '%s' and '%s' and SHIFT_ID='%s' and STATION_ID_CID_TRIGGER='%s'" ("condition")) -> (w553:string)
                            n79 = Format Into String(format string=w553, w546, w545, w551, w548) -> (resulting string=w552:string)  [unwired: 2 in, 1 out]
                          }
                          frame "3" {
                            w559 = "6" ("input 3")
                            n80 = Concatenate Strings("select PLAN_DATE from " ("string"), w558, "\n" ("string"), "Where PLAN_DATE between '%s' and '%s' and SHIFT_ID='%s' and STATION_ID_CID_TRIGGER='%s'   " ("condition")) -> (w564:string)
                            n81 = Format Into String(format string=w564, w557, w556, w562, w559) -> (resulting string=w563:string)  [unwired: 2 in, 1 out]
                          }
                        }
                      }
                    }
                  }
                  frame Enabled {
                    n82 = case shown="\"ST 4\"" w566 {
                      tunnel: ["1" "2" "3" "4" "5" "6" "1"] -> w573
                      frame "ST 1" {
                      }
                      frame "ST 2" {
                      }
                      frame "ST 3" {
                      }
                      frame "ST 4" {
                      }
                      frame "ST 5" {
                      }
                      frame "ST 6" {
                      }
                      frame "ALL", Default {
                      }
                    }
                    n83 = Equal?(x=w570, y="ALL" ("condition")) -> (x = y?=w572:bool)
                    n84 = Select(t="", s=w572, f=" and SHIFT_ID='%s'" ("condition")) -> (s? t:f=w574:string)
                    n85 = Concatenate Strings("select PLAN_DATE from STATION_" ("string"), w573, "_LOG_HISTORY\nWhere PLAN_DATE between '%s' and '%s' and STATION_ID_CID_TRIGGER=" ("condition"), w573, w574) -> (w579:string)
                    n86 = case shown="True" w572 {
                      tunnel: w579 -> [w582 w589]
                      tunnel: [w585 w588] -> w571
                      tunnel: w570 -> [w581 _]
                      tunnel: w569 -> [w584 w587]
                      tunnel: w568 -> [w583 w586]
                      frame False {
                        n87 = Format Into String(format string=w582, w584, w583, w581) -> (resulting string=w585:string)  [unwired: 2 in, 1 out]
                      }
                      frame True {
                        n88 = Format Into String(format string=w589, w587, w586) -> (resulting string=w588:string)  [unwired: 2 in, 1 out]
                      }
                    }
                  }
                }
                n89 = local read "Select Station"() -> (w121:string)
                n90 = local read "Shift"() -> (w47:string)
                n91 = call "BREAKDOWN_FOR_DAYWISE_FINAL.vi"("Shift"=w47, "Select Line 2"=w121) -> ("String"=w109:string, "All Station String"=w62:string[])  [unwired: 5 in, 3 out]
                n92 = call "Execute query.vi"("error in (no error)"=w192, "String"=w197, "connection reference"=w120) -> ("error out"=w54:errorcluster, "Table"=w195:string[][], "connection reference 2"=w185:T2)  [unwired: 5 in, 1 out]
                n93 = case shown="\"ST 6\"" "Select Station" {
                  tunnel: [_ "1" "2" "3" "4" "5" "6"] -> w113
                  frame "ALL", Default {
                  }
                  frame "ST 1" {
                  }
                  frame "ST 2" {
                  }
                  frame "ST 3" {
                  }
                  frame "ST 4" {
                  }
                  frame "ST 5" {
                  }
                  frame "ST 6" {
                  }
                }
                n94 = Index Array(array=w195, index (col) #1=0 ("disabled index (col)"), index (col) #2=2 ("index (col)")) -> (element #1=w196:string[], element #2=w188:string[])  [unwired: 2 in]
                n95 = call "Timestamp to string.vi"("time stamp"="From") -> ("Date"=w50:string)  [unwired: 8 in, 2 out]
                n96 = call "Timestamp to string.vi"("time stamp"="To") -> ("Date"=w48:string)  [unwired: 8 in, 2 out]
                n97 = call "Search_1d_array_element.vi"("BD Date"=w196) -> ("Count out"=→"Count out":string[], "Elements Found out"=w143:string[])  [unwired: 6 in, 1 out]
                "Elements Found out" <- w143
                n98 = call "Search_1d_array_element.vi"("BD Date"=w188) -> ("Count out"=→"Count":string[], "Elements Found out"=→"Station ID":string[])  [unwired: 6 in, 1 out]
                n99 = Equal?(x=w47, y="ALL") -> (x = y?=w110:bool)
                n100 = flat-sequence {
                  tunnel: w54 -> [w609]
                  tunnel: w185 -> [w629]
                  tunnel: [w627] -> w184
                  tunnel: [w626] -> w183
                  tunnel: [w625] -> w182
                  tunnel: [w610] -> w181
                  tunnel: w143 -> [w623]
                  tunnel: [w623] -> w142
                  tunnel: w113 -> [w621]
                  tunnel: [w621] -> w138
                  tunnel: w109 -> [w622]
                  tunnel: [w622] -> w136
                  tunnel: w47 -> [w620]
                  tunnel: [w619] -> w132
                  tunnel: w47 -> [w619]
                  tunnel: w110 -> [w617]
                  tunnel: [w617] -> w127
                  tunnel: w50 -> [w616]
                  tunnel: w48 -> [w615]
                  tunnel: [w614] -> w108
                  tunnel: w50 -> [w614]
                  tunnel: [w613] -> w107
                  tunnel: w48 -> [w613]
                  tunnel: [w612] -> w63
                  tunnel: w62 -> [w612]
                  tunnel: [w611] -> w57
                  tunnel: w50 -> [w611]
                  tunnel: w184 -> [w659]
                  tunnel: w183 -> [w654]
                  tunnel: w182 -> [w655]
                  tunnel: w181 -> [w658]
                  tunnel: [w655] -> w180
                  tunnel: [w654] -> w179
                  tunnel: [w653] -> w178
                  tunnel: [w652] -> w177
                  tunnel: [w651] -> w176
                  tunnel: [w650] -> w175
                  tunnel: w142 -> [w649]
                  tunnel: [w649] -> w141
                  tunnel: w138 -> [w648]
                  tunnel: [w648] -> w137
                  tunnel: w136 -> [w647]
                  tunnel: [w647] -> w135
                  tunnel: w132 -> [w646]
                  tunnel: [w646] -> w131
                  tunnel: w127 -> [w645]
                  tunnel: [w645] -> w126
                  tunnel: w108 -> [w644]
                  tunnel: w107 -> [w643]
                  tunnel: [w644] -> w106
                  tunnel: [w643] -> w105
                  tunnel: [w642] -> w64
                  tunnel: w63 -> [w642]
                  tunnel: [w641] -> w58
                  tunnel: w57 -> [w641]
                  tunnel: w180 -> [w693]
                  tunnel: w179 -> [w692]
                  tunnel: w178 -> [w691]
                  tunnel: w177 -> [w690]
                  tunnel: w176 -> [w687]
                  tunnel: w175 -> [w686]
                  tunnel: [w693] -> w174
                  tunnel: [w692] -> w173
                  tunnel: [w691] -> w172
                  tunnel: [w690] -> w171
                  tunnel: [w685] -> w170
                  tunnel: [w684] -> w169
                  tunnel: [w683] -> w168
                  tunnel: [w682] -> w167
                  tunnel: w141 -> [w681]
                  tunnel: [w681] -> w140
                  tunnel: w137 -> [w677]
                  tunnel: w135 -> [w676]
                  tunnel: [w676] -> w134
                  tunnel: w131 -> [w680]
                  tunnel: [w680] -> w130
                  tunnel: w126 -> [w678]
                  tunnel: [w678] -> w125
                  tunnel: [w677] -> w124
                  tunnel: w106 -> [w675]
                  tunnel: w105 -> [w674]
                  tunnel: [w675] -> w104
                  tunnel: [w674] -> w103
                  tunnel: [w673] -> w65
                  tunnel: w64 -> [w673]
                  tunnel: [w672] -> w59
                  tunnel: w58 -> [w672]
                  tunnel: w174 -> [w728]
                  tunnel: w173 -> [w727]
                  tunnel: w172 -> [w726]
                  tunnel: w171 -> [w725]
                  tunnel: w170 -> [w724]
                  tunnel: w169 -> [w723]
                  tunnel: w168 -> [w720]
                  tunnel: w167 -> [w719]
                  tunnel: [w728] -> w166
                  tunnel: [w727] -> w165
                  tunnel: [w726] -> w164
                  tunnel: [w725] -> w163
                  tunnel: [w724] -> w162
                  tunnel: [w723] -> w161
                  tunnel: [w718] -> w160
                  tunnel: [w717] -> w159
                  tunnel: [w716] -> w158
                  tunnel: [w715] -> w157
                  tunnel: w140 -> [w714]
                  tunnel: [w714] -> w139
                  tunnel: w134 -> [w711]
                  tunnel: [w711] -> w133
                  tunnel: w130 -> [w713]
                  tunnel: [w713] -> w129
                  tunnel: w125 -> [w709]
                  tunnel: w124 -> [w710]
                  tunnel: [w710] -> w123
                  tunnel: [w709] -> w122
                  tunnel: w104 -> [w708]
                  tunnel: w103 -> [w707]
                  tunnel: [w708] -> w102
                  tunnel: [w707] -> w101
                  tunnel: w65 -> [w706]
                  tunnel: [w706] -> w60
                  tunnel: w59 -> [w705]
                  tunnel: [w705] -> w55
                  tunnel: w166 -> [w765]
                  tunnel: w165 -> [w764]
                  tunnel: w164 -> [w763]
                  tunnel: w163 -> [w762]
                  tunnel: w162 -> [w761]
                  tunnel: w161 -> [w760]
                  tunnel: w160 -> [w759]
                  tunnel: w159 -> [w758]
                  tunnel: w158 -> [w755]
                  tunnel: w157 -> [w754]
                  tunnel: [w765] -> w92
                  tunnel: [w764] -> w90
                  tunnel: [w763] -> w88
                  tunnel: [w762] -> w86
                  tunnel: [w761] -> w84
                  tunnel: [w760] -> w82
                  tunnel: [w759] -> w80
                  tunnel: [w758] -> w78
                  tunnel: [w753] -> w76
                  tunnel: [w752] -> w74
                  tunnel: [w751] -> w72
                  tunnel: [w750] -> w70
                  tunnel: w139 -> [w749]
                  tunnel: [w749] -> w68
                  tunnel: w133 -> [w742]
                  tunnel: w129 -> [w747]
                  tunnel: w123 -> [w746]
                  tunnel: w122 -> [w743]
                  tunnel: w102 -> [w745]
                  tunnel: w101 -> [w744]
                  tunnel: [w743] -> w66
                  tunnel: [w741] -> w61
                  tunnel: w60 -> [w741]
                  tunnel: [w740] -> w56
                  tunnel: w55 -> [w740]
                  tunnel: w92 -> [w792]
                  tunnel: [w792] -> w91
                  tunnel: w90 -> [w791]
                  tunnel: [w791] -> w89
                  tunnel: w88 -> [w790]
                  tunnel: [w790] -> w87
                  tunnel: w86 -> [w789]
                  tunnel: [w789] -> w85
                  tunnel: w84 -> [w788]
                  tunnel: [w788] -> w83
                  tunnel: w82 -> [w787]
                  tunnel: [w787] -> w81
                  tunnel: w80 -> [w786]
                  tunnel: [w786] -> w79
                  tunnel: w78 -> [w785]
                  tunnel: [w785] -> w77
                  tunnel: w76 -> [w784]
                  tunnel: [w784] -> w75
                  tunnel: w74 -> [w783]
                  tunnel: [w783] -> w73
                  tunnel: w72 -> [w782]
                  tunnel: [w782] -> w71
                  tunnel: w70 -> [w781]
                  tunnel: [w781] -> w69
                  tunnel: w68 -> [w780]
                  tunnel: [w780] -> w67
                  tunnel: w66 -> [w779]
                  tunnel: w61 -> [w778]
                  tunnel: w56 -> [w777]
                  tunnel: w91 -> [w836]
                  tunnel: w89 -> [w813]
                  tunnel: w87 -> [w812]
                  tunnel: w85 -> [w835]
                  tunnel: w83 -> [w811]
                  tunnel: w81 -> [w834]
                  tunnel: w79 -> [w810]
                  tunnel: w77 -> [w833]
                  tunnel: w75 -> [w809]
                  tunnel: w73 -> [w832]
                  tunnel: w71 -> [w837]
                  tunnel: w69 -> [w838]
                  tunnel: [w847] -> w156
                  tunnel: [w813] -> w155
                  tunnel: [w846] -> w154
                  tunnel: [w812] -> w153
                  tunnel: [w845] -> w152
                  tunnel: [w811] -> w151
                  tunnel: [w844] -> w150
                  tunnel: [w810] -> w149
                  tunnel: [w843] -> w148
                  tunnel: [w809] -> w147
                  tunnel: [w842] -> w146
                  tunnel: [w841] -> w145
                  tunnel: [w840] -> w144
                  tunnel: w67 -> [w839]
                  tunnel: [w839] -> w128
                  tunnel: [w838] -> w117
                  tunnel: [w837] -> w115
                  tunnel: [w836] -> w98
                  tunnel: [w835] -> w97
                  tunnel: [w834] -> w96
                  tunnel: [w833] -> w95
                  tunnel: [w832] -> w94
                  tunnel: [w830] -> w93
                  tunnel: [w819] -> w46
                  tunnel: [w818] -> w45
                  tunnel: [w817] -> w44
                  tunnel: [w816] -> w43
                  tunnel: [w815] -> w42
                  tunnel: [w814] -> w41
                  tunnel: w156 -> [w925]
                  tunnel: w155 -> [w924]
                  tunnel: w154 -> [w895]
                  tunnel: w153 -> [w923]
                  tunnel: w152 -> [w894]
                  tunnel: w151 -> [w922]
                  tunnel: w150 -> [w893]
                  tunnel: w149 -> [w921]
                  tunnel: w148 -> [w892]
                  tunnel: w147 -> [w920]
                  tunnel: w146 -> [w891]
                  tunnel: w145 -> [w918]
                  tunnel: w144 -> [w919]
                  tunnel: w128 -> [_]
                  tunnel: [w897] -> w118
                  tunnel: w117 -> [w897]
                  tunnel: [w896] -> w116
                  tunnel: w115 -> [w896]
                  tunnel: w98 -> [w890]
                  tunnel: w97 -> [w889]
                  tunnel: w96 -> [w888]
                  tunnel: w95 -> [w887]
                  tunnel: w94 -> [w886]
                  tunnel: w93 -> [w885]
                  tunnel: w46 -> [w870]
                  tunnel: w45 -> [w864]
                  tunnel: w44 -> [w863]
                  tunnel: w43 -> [w862]
                  tunnel: w42 -> [w861]
                  tunnel: w41 -> [w860]
                  frame #0 {
                    n101 = case shown="False" w617 {
                      tunnel: w622 -> [w633 w639]
                      tunnel: w621 -> [_ _]
                      tunnel: w620 -> [_ w638]
                      tunnel: [w632 w637] -> w618
                      tunnel: w616 -> [w631 w636]
                      tunnel: w615 -> [w630 w635]
                      frame True {
                        n102 = Format Into String(format string=w633, w631, w630, 1 ("BREAKDOWN_STK_HOLD_ID")) -> (resulting string=w632:string)  [unwired: 2 in, 1 out]
                      }
                      frame False {
                        n103 = Format Into String(format string=w639, w636, w635, 1 ("BREAKDOWN_STK_HOLD_ID"), w638) -> (resulting string=w637:string)  [unwired: 2 in, 1 out]
                      }
                    }
                    n104 = call "Execute query.vi"("error in (no error)"=w609, "String"=w618, "connection reference"=w629) -> ("error out"=w624:errorcluster, "Table"=w628:string[][], "connection reference 2"=w627:T2)  [unwired: 5 in, 1 out]
                    n105 = call "DAYwise_bd_summery_FINAL.vi"("O/P 3"=w623, "error in (no error)"=w624, "Table"=w628) -> ("error out"=w610:errorcluster, "O/P 2"=w626:string[], "O/P"=w625:string[])  [unwired: 6 in]
                  }
                  frame #1 {
                    n106 = case shown="False" w645 {
                      tunnel: [w664 w670] -> w657
                      tunnel: w648 -> [_ _]
                      tunnel: w647 -> [w663 w669]
                      tunnel: w646 -> [_ w668]
                      tunnel: w644 -> [w662 w667]
                      tunnel: w643 -> [w661 w666]
                      frame True {
                        n107 = Format Into String(format string=w663, w662, w661, 2 ("BREAKDOWN_STK_HOLD_ID")) -> (resulting string=w664:string)  [unwired: 2 in, 1 out]
                      }
                      frame False {
                        n108 = Format Into String(format string=w669, w667, w666, 2 ("BREAKDOWN_STK_HOLD_ID"), w668) -> (resulting string=w670:string)  [unwired: 2 in, 1 out]
                      }
                    }
                    n109 = call "Execute query.vi"("error in (no error)"=w658, "String"=w657, "connection reference"=w659) -> ("error out"=w660:errorcluster, "Table"=w656:string[][], "connection reference 2"=w651:T2)  [unwired: 5 in, 1 out]
                    n110 = call "DAYwise_bd_summery_FINAL.vi"("O/P 3"=w649, "error in (no error)"=w660, "Table"=w656) -> ("error out"=w650:errorcluster, "O/P 2"=w653:string[], "O/P"=w652:string[])  [unwired: 6 in]
                  }
                  frame #2 {
                    n111 = case shown="False" w678 {
                      tunnel: [w697 w703] -> w679
                      tunnel: w677 -> [_ _]
                      tunnel: w680 -> [_ w702]
                      tunnel: w676 -> [w696 w701]
                      tunnel: w675 -> [w695 w700]
                      tunnel: w674 -> [w694 w699]
                      frame True {
                        n112 = Format Into String(format string=w696, w695, w694, 3 ("BREAKDOWN_STK_HOLD_ID")) -> (resulting string=w697:string)  [unwired: 2 in, 1 out]
                      }
                      frame False {
                        n113 = Format Into String(format string=w701, w700, w699, 3 ("BREAKDOWN_STK_HOLD_ID"), w702) -> (resulting string=w703:string)  [unwired: 2 in, 1 out]
                      }
                    }
                    n114 = call "Execute query.vi"("error in (no error)"=w686, "String"=w679, "connection reference"=w687) -> ("error out"=w688:errorcluster, "Table"=w689:string[][], "connection reference 2"=w682:T2)  [unwired: 5 in, 1 out]
                    n115 = call "DAYwise_bd_summery_FINAL.vi"("O/P 3"=w681, "error in (no error)"=w688, "Table"=w689) -> ("error out"=w683:errorcluster, "O/P 2"=w685:string[], "O/P"=w684:string[])  [unwired: 6 in]
                  }
                  frame #3 {
                    n116 = case shown="False" w709 {
                      tunnel: [w732 w738] -> w712
                      tunnel: w713 -> [_ w737]
                      tunnel: w710 -> [_ _]
                      tunnel: w711 -> [w731 w736]
                      tunnel: w708 -> [w730 w735]
                      tunnel: w707 -> [w729 w734]
                      frame True {
                        n117 = Format Into String(format string=w731, w730, w729, 4 ("BREAKDOWN_STK_HOLD_ID")) -> (resulting string=w732:string)  [unwired: 2 in, 1 out]
                      }
                      frame False {
                        n118 = Format Into String(format string=w736, w735, w734, 4 ("BREAKDOWN_STK_HOLD_ID"), w737) -> (resulting string=w738:string)  [unwired: 2 in, 1 out]
                      }
                    }
                    n119 = call "Execute query.vi"("error in (no error)"=w720, "String"=w712, "connection reference"=w719) -> ("error out"=w722:errorcluster, "Table"=w721:string[][], "connection reference 2"=w715:T2)  [unwired: 5 in, 1 out]
                    n120 = call "DAYwise_bd_summery_FINAL.vi"("O/P 3"=w714, "error in (no error)"=w722, "Table"=w721) -> ("error out"=w716:errorcluster, "O/P 2"=w718:string[], "O/P"=w717:string[])  [unwired: 6 in]
                  }
                  frame #4 {
                    n121 = case shown="False" w743 {
                      tunnel: [w769 w775] -> w748
                      tunnel: w747 -> [_ w774]
                      tunnel: w742 -> [w768 w773]
                      tunnel: w746 -> [_ _]
                      tunnel: w745 -> [w767 w772]
                      tunnel: w744 -> [w766 w771]
                      frame True {
                        n122 = Format Into String(format string=w768, w767, w766, 5 ("BREAKDOWN_STK_HOLD_ID")) -> (resulting string=w769:string)  [unwired: 2 in, 1 out]
                      }
                      frame False {
                        n123 = Format Into String(format string=w773, w772, w771, 5 ("BREAKDOWN_STK_HOLD_ID"), w774) -> (resulting string=w775:string)  [unwired: 2 in, 1 out]
                      }
                    }
                    n124 = call "Execute query.vi"("error in (no error)"=w755, "String"=w748, "connection reference"=w754) -> ("error out"=w756:errorcluster, "Table"=w757:string[][], "connection reference 2"=w751:T2)  [unwired: 5 in, 1 out]
                    n125 = call "DAYwise_bd_summery_FINAL.vi"("O/P 3"=w749, "error in (no error)"=w756, "Table"=w757) -> ("error out"=w750:errorcluster, "O/P 2"=w753:string[], "O/P"=w752:string[])  [unwired: 6 in]
                  }
                  frame #5 {
                    n126 = disable-structure shown="Disabled" {
                      disable-tunnel: w779 -> [w796 _]
                      disable-tunnel: w778 -> [w795 _]
                      disable-tunnel: w777 -> [w793 _]
                      frame Disabled {
                        n127 = local read "Shift"() -> (w794:string)
                        n128 = for {
                          tunnel: w796 -> [w801]
                          tunnel: w795 -> [w800] mode=indexing
                          tunnel: w794 -> [w799]
                          tunnel: w793 -> [w798]
                          n129 = case shown="False" w801 {
                            tunnel: [w804 w808] -> w797
                            tunnel: w800 -> [w803 w807]
                            tunnel: w799 -> [_ w806]
                            tunnel: w798 -> [w802 w805]
                            frame True {
                              n130 = Format Into String(format string=w803, w802) -> (resulting string=w804:string)  [unwired: 2 in, 1 out]
                            }
                            frame False {
                              n131 = Format Into String(format string=w807, w805, w806) -> (resulting string=w808:string)  [unwired: 2 in, 1 out]
                            }
                          }
                          n132 = call "Execute query.vi"("String"=w797) -> ()  [unwired: 7 in, 4 out]
                        }
                      }
                      frame Enabled {
                      }
                    }
                  }
                  frame #6 {
                    n133 = call "String to numeric.vi"("Array"=w836) -> ("Array 2"=w818:dbl[])  [unwired: 4 in]
                    n134 = call "String to numeric.vi"("Array"=w835) -> ("Array 2"=w817:dbl[])  [unwired: 4 in]
                    n135 = call "String to numeric.vi"("Array"=w834) -> ("Array 2"=w816:dbl[])  [unwired: 4 in]
                    n136 = call "String to numeric.vi"("Array"=w833) -> ("Array 2"=w815:dbl[])  [unwired: 4 in]
                    n137 = call "String to numeric.vi"("Array"=w832) -> ("Array 2"=w814:dbl[])  [unwired: 4 in]
                    n138 = Decimal String To Number(string=w813) -> (number=w829:i32[])  [unwired: 2 in, 1 out]
                    n139 = Decimal String To Number(string=w812) -> (number=w828:i32[])  [unwired: 2 in, 1 out]
                    n140 = Decimal String To Number(string=w811) -> (number=w827:i32[])  [unwired: 2 in, 1 out]
                    n141 = Decimal String To Number(string=w810) -> (number=w826:i32[])  [unwired: 2 in, 1 out]
                    n142 = Decimal String To Number(string=w809) -> (number=w825:i32[])  [unwired: 2 in, 1 out]
                    n143 = Compound Arithmetic op=ADD(w818, w817, w816, w815, w814) -> (w831:dbl[])
                    n144 = for {
                      tunnel: w831 -> [w857] mode=indexing
                      tunnel: [w856] -> w830 mode=indexing
                      n145 = Format Value(format string="%<%H:%M:%S>t", value (0)=w857) -> (output string=w856:string)  [unwired: 1 in]
                    }
                    n146 = Add Array Elements(numeric array=w829) -> (sum=w824:i32)
                    n147 = Add Array Elements(numeric array=w828) -> (sum=w823:i32)
                    n148 = Add Array Elements(numeric array=w827) -> (sum=w822:i32)
                    n149 = Add Array Elements(numeric array=w826) -> (sum=w821:i32)
                    n150 = Add Array Elements(numeric array=w825) -> (sum=w820:i32)
                    n151 = Build Array(w836) -> (w855:string[][])
                    n152 = Build Array(w835) -> (w854:string[][])
                    n153 = Build Array(w834) -> (w853:string[][])
                    n154 = Build Array(w833) -> (w852:string[][])
                    n155 = Build Array(w832) -> (w851:string[][])
                    n156 = Build Array(w839) -> (w848:string[][])
                    n157 = Compound Arithmetic op=ADD(w829, w828, w827, w826, w825) -> (w849:i32[])
                    n158 = Transpose 2D Array(2D array=w855) -> (transposed array=w846:string[][])
                    n159 = Transpose 2D Array(2D array=w854) -> (transposed array=w845:string[][])
                    n160 = Transpose 2D Array(2D array=w853) -> (transposed array=w844:string[][])
                    n161 = Transpose 2D Array(2D array=w852) -> (transposed array=w843:string[][])
                    n162 = Transpose 2D Array(2D array=w851) -> (transposed array=w842:string[][])
                    n163 = Transpose 2D Array(2D array=w848) -> (transposed array=w847:string[][])
                    n164 = Build Array(w830) -> (w850:string[][])
                    n165 = Number To Decimal String(number=w849) -> (decimal integer string=w841:string[])  [unwired: 1 in]
                    n166 = Build Array(w824, w823, w822, w821, w820) -> (w819:i32[])
                    n167 = Transpose 2D Array(2D array=w850) -> (transposed array=w840:string[][])
                  }
                  frame #7 {
                    n168 = Insert Into Array(array=w925, index (col)=1 ("disabled index (col)"), new element #1=w924, new element #2=w895, new element #3=w923, new element #4=w894, new element #5=w922, new element #6=w893, new element #7=w921, new element #8=w892, new element #9=w920, new element #10=w891, new element #11=w918, new element #12=w919) -> (w917:string[][])  [unwired: 1 in]
                    "Table Control" <- w917
                    n169 = disable-structure shown="Enabled" {
                      disable-tunnel: w890 -> [w951 w968]
                      disable-tunnel: w889 -> [w950 w966]
                      disable-tunnel: w888 -> [w949 w965]
                      disable-tunnel: w887 -> [w948 w964]
                      disable-tunnel: w886 -> [w947 w963]
                      disable-tunnel: w885 -> [w945 w962]
                      disable-tunnel: [w932 w967] -> w884
                      disable-tunnel: [w931 w957] -> w883
                      disable-tunnel: [w930 w958] -> w882
                      disable-tunnel: [w929 w959] -> w881
                      disable-tunnel: [w928 w960] -> w880
                      disable-tunnel: [w927 w961] -> w879
                      frame Disabled {
                        n170 = Fract/Exp String To Number(string=w951) -> (number=w956:dbl[])  [unwired: 3 in, 1 out]
                        n171 = Fract/Exp String To Number(string=w950) -> (number=w955:dbl[])  [unwired: 3 in, 1 out]
                        n172 = Fract/Exp String To Number(string=w949) -> (number=w954:dbl[])  [unwired: 3 in, 1 out]
                        n173 = Fract/Exp String To Number(string=w948) -> (number=w953:dbl[])  [unwired: 3 in, 1 out]
                        n174 = Fract/Exp String To Number(string=w947) -> (number=w952:dbl[])  [unwired: 3 in, 1 out]
                        n175 = Fract/Exp String To Number(string=w945) -> (number=w946:dbl[])  [unwired: 3 in, 1 out]
                        n176 = Add Array Elements(numeric array=w956) -> (sum=w938:dbl)
                        n177 = Add Array Elements(numeric array=w955) -> (sum=w937:dbl)
                        n178 = Add Array Elements(numeric array=w954) -> (sum=w936:dbl)
                        n179 = Add Array Elements(numeric array=w953) -> (sum=w935:dbl)
                        n180 = Add Array Elements(numeric array=w952) -> (sum=w934:dbl)
                        n181 = Add Array Elements(numeric array=w946) -> (sum=w933:dbl)
                        n182 = Number To Fractional String(number=w937, precision (6)=i16 2) -> (F-format string=w931:string)  [unwired: 2 in]
                        n183 = Number To Fractional String(number=w938, precision (6)=i16 2) -> (F-format string=w932:string)  [unwired: 2 in]
                        n184 = Number To Fractional String(number=w936, precision (6)=i16 2) -> (F-format string=w930:string)  [unwired: 2 in]
                        n185 = Number To Fractional String(number=w935, precision (6)=i16 2) -> (F-format string=w929:string)  [unwired: 2 in]
                        n186 = Number To Fractional String(number=w934, precision (6)=i16 2) -> (F-format string=w928:string)  [unwired: 2 in]
                        n187 = Number To Fractional String(number=w933, precision (6)=i16 2) -> (F-format string=w927:string)  [unwired: 2 in]
                      }
                      frame Enabled {
                        n188 = call "time string to minutes string.vi"("Array"=w968) -> ("output string"=w967:string)  [unwired: 10 in]
                        n189 = call "time string to minutes string.vi"("Array"=w966) -> ("output string"=w957:string)  [unwired: 10 in]
                        n190 = call "time string to minutes string.vi"("Array"=w965) -> ("output string"=w958:string)  [unwired: 10 in]
                        n191 = call "time string to minutes string.vi"("Array"=w964) -> ("output string"=w959:string)  [unwired: 10 in]
                        n192 = call "time string to minutes string.vi"("Array"=w962) -> ("output string"=w961:string)  [unwired: 10 in]
                        n193 = call "time string to minutes string.vi"("Array"=w963) -> ("output string"=w960:string)  [unwired: 10 in]
                      }
                    }
                    n194 = Add Array Elements(numeric array=w864) -> (sum=w865:dbl)
                    n195 = Add Array Elements(numeric array=w863) -> (sum=w866:dbl)
                    n196 = Add Array Elements(numeric array=w862) -> (sum=w867:dbl)
                    n197 = Add Array Elements(numeric array=w861) -> (sum=w868:dbl)
                    n198 = Add Array Elements(numeric array=w860) -> (sum=w869:dbl)
                    n199 = Build Array(w865, w866, w867, w868, w869) -> (w859:dbl[])
                    n200 = Index Array(array=w917, index (col) #1=1 ("disabled index (col)")) -> (element #1=w915:string[], element #3=w914:string[], element #5=w913:string[], element #7=w912:string[], element #9=w911:string[], element #11=w910:string[])  [unwired: 23 in, 6 out]
                    n201 = call "SUM_ARRAY.vi"("Array"=w915) -> ("F-format string"=w909:string)  [unwired: 6 in]
                    n202 = call "SUM_ARRAY.vi"("Array"=w914) -> ("F-format string"=w908:string)  [unwired: 6 in]
                    n203 = call "SUM_ARRAY.vi"("Array"=w913) -> ("F-format string"=w907:string)  [unwired: 6 in]
                    n204 = call "SUM_ARRAY.vi"("Array"=w912) -> ("F-format string"=w906:string)  [unwired: 6 in]
                    n205 = call "SUM_ARRAY.vi"("Array"=w911) -> ("F-format string"=w905:string)  [unwired: 6 in]
                    n206 = call "SUM_ARRAY.vi"("Array"=w910) -> ("F-format string"=w904:string)  [unwired: 6 in]
                    n207 = call "CONCATINATE_STRING.vi"("F-format string"=w884, "F-format string 2"=w909) -> ("concatenated string"=→"S":string)  [unwired: 9 in]
                    n208 = call "CONCATINATE_STRING.vi"("F-format string"=w883, "F-format string 2"=w908) -> ("concatenated string"=→"Mat":string)  [unwired: 9 in]
                    n209 = call "CONCATINATE_STRING.vi"("F-format string"=w882, "F-format string 2"=w907) -> ("concatenated string"=→"Maint":string)  [unwired: 9 in]
                    n210 = call "CONCATINATE_STRING.vi"("F-format string"=w881, "F-format string 2"=w906) -> ("concatenated string"=→"Q":string)  [unwired: 9 in]
                    n211 = call "CONCATINATE_STRING.vi"("F-format string"=w880, "F-format string 2"=w905) -> ("concatenated string"=→"SS":string)  [unwired: 9 in]
                    n212 = call "CONCATINATE_STRING.vi"("F-format string"=w879, "F-format string 2"=w904) -> ("concatenated string"=→"T":string)  [unwired: 9 in]
                    n213 = call "Plot PieChart.vi"("Label"=string[] ["Safety", "Material", "Maintenance", "Quality", "Startup_Setup"]) -> ("Labelling"=w874:cluster{dbl, "String":string}[])  [unwired: 10 in]
                    n214 = property on="Duration" class="3D Pie (strict)"("Plot Specific:Color and Name"=w874) -> (error out=w876:errorcluster)  [unwired: 2 in, 1 out]
                    n215 = property on="Count" class="3D Pie (strict)"("Plot Specific:Color and Name"=w874) -> (error out=w873:errorcluster)  [unwired: 2 in, 1 out]
                    n216 = call-poly <vilib>:"Plot Helper.vi"("x vector"=w859) -> ("error out"=w878:errorcluster, "3D Plot lvclass Array out"=→"Duration":refnum<class "3D Plot Datatype.lvclass">[])  [unwired: 2 in, 7 out]
                    n217 = call-poly <vilib>:"Plot Helper.vi"("x vector"=w870) -> ("error out"=w872:errorcluster, "3D Plot lvclass Array out"=→"Count":refnum<class "3D Plot Datatype.lvclass">[])  [unwired: 2 in, 7 out]
                    n218 = Unbundle By Name(w876) -> ()  [unwired: 1 out]
                    n219 = Unbundle By Name(w873) -> ()  [unwired: 1 out]
                    n220 = Unbundle By Name(w878) -> ()  [unwired: 1 out]
                    n221 = Unbundle By Name(w872) -> ()  [unwired: 1 out]
                    "O/P 4" <- w924
                  }
                }
              }
            }
          }
        }
        "error out 2" <- w33
        "Boolean" <- "Get Rport 2"
      }
      event "Download 2": Value Change {
        n222 = event-data() -> ()  [unwired: 1 in, 6 out]
        n223 = local read "Table Control"() -> (w982:string[][])
        n224 = Empty Array?(array=w982) -> (empty?=w983:bool)
        n225 = case shown="False" w983 {
          tunnel: w985 -> [w1003 w1012]
          tunnel: [w1002 w1012] -> w984
          tunnel: w982 -> [w988 _]
          frame False {
            w997 = 1 ("index (row)")
            n226 = local read "Select Station"() -> (w994:string)
            n227 = local read "From"() -> (w990:timestamp)
            n228 = local read "To"() -> (w989:timestamp)
            n229 = case shown="\"ALL\", Default" w994 {
              tunnel: ["All" "250T-3" "250T-2" "250T-1" "400T-1" "150T-1" "400T-2"] -> w993
              frame "ALL", Default {
              }
              frame "ST 1" {
              }
              frame "ST 2" {
              }
              frame "ST 3" {
              }
              frame "ST 4" {
              }
              frame "ST 5" {
              }
              frame "ST 6" {
              }
            }
            n230 = call "Timestamp to string.vi"("time stamp"=w990) -> ("Date"=w992:string)  [unwired: 8 in, 2 out]
            n231 = call "Timestamp to string.vi"("time stamp"=w989) -> ("Date"=w991:string)  [unwired: 8 in, 2 out]
            n232 = local read "Shift"() -> (w995:string)
            n233 = Replace Array Subset(array=string[][] [["L&L Products", "Breakdown Summary", "Daywise", "", "", "", "", "", "", "", "", "", ""], ["From:", "", "To:", "", "Station:", "", "Shift:", "", "", "", "", "", ""], ["", "", "", "", "", "", "", "", "", "", "", "", ""], ["Date", "Safety Count", "Duration", "Material Count", "Duration", "Maintenance Count", "Duration", "Quality Count", "Duration", "Startup_Setup Count", "Duration", "Total Count", "Duration"]] ("Column Header Strings[]"), new element #1=w992, index (row) #1=w997, index (col) #1=w997, new element #2=w991, index (row) #2=w997, index (col) #2=3 ("disabled index (col)"), new element #3=w993, index (row) #3=w997, index (col) #3=5 ("disabled index (col)"), new element #4=w995, index (row) #4=w997, index (col) #4=7 ("disabled index (col)")) -> (w1000:string[][])
            n234 = call "Download_Report_subvi.vi"("error in (no error)"=w1003, "Value"=w988, "Column Header Strings[]"=w1000) -> ("error out"=w1002:errorcluster)  [unwired: 8 in]
          }
          frame True {
            n235 = One Button Dialog(message="No record found!") -> ()  [unwired: 1 in, 1 out]
          }
        }
      }
      event "Cancel Button - Archive": Value Change {
        n236 = event-data() -> ()  [unwired: 1 in, 6 out]
      }
    }
    n237 = Wait (ms)(milliseconds to wait=u32 50) -> ()  [unwired: 1 out]
  }
  n238 = Concatenate Strings("select * from " ("string"), "STATION_1_LOG_HISTORY" ("table"), "\n" ("string"), "Where month(BREAKDOWN_DATE) ='%s' and  BREAKDOWN_STK_HOLD_ID ='%d' and  STATION_ID_CID_TRIGGER='%s' and SHIFT_ID='%s'\n" ("condition")) -> ()  [unwired: 1 out]
  n239 = call <vilib>:"DB Tools Close Connection.vi"("error in (no error)"=w5, "connection reference"=w6) -> ("error out"=w4:errorcluster)  [unwired: 5 in]
  n240 = call <vilib>:"Clear Errors.vi"("error in (no error)"=w4) -> ("error out"=w10:errorcluster)  [unwired: 5 in, 1 out]
  n241 = property class="App"(error in=w10) -> (error out=w9:errorcluster, "App.Kind"=w8:T3)  [unwired: 1 in, 1 out]
  n242 = case shown="\"Development System\", Default" w8 {
    tunnel: w9 -> [w1017 w1022]
    tunnel: [w1016 w1021] -> w7
    frame "Development System", Default {
      n243 = disable-structure shown="Enabled" {
        disable-tunnel: w1017 -> [w1019 w1020]
        disable-tunnel: [w1018 w1020] -> w1016
        frame Enabled {
          n244 = invoke class="VI" method="FP.Close"(error in=w1019) -> (error out=w1018:errorcluster)  [unwired: 2 in, 2 out]
        }
        frame Disabled {
        }
      }
    }
    frame "Run Time System" {
      n245 = invoke class="VI" method="FP.Close"(error in=w1022) -> (error out=w1021:errorcluster)  [unwired: 2 in, 2 out]
    }
  }
  "error out" <- w7
